vi "Curtin_SaveToExcel.vi"(8 "plots":refnum<vi>[](array[refnum])) -> ()   [LabVIEW 2022 SP3]
uses:
  <vilib>/express/express shared/NI_ExcelFile/Ctrls/FileOperation.ctl
  <vilib>/express/express shared/NI_ExcelFile/SubVIs/WriteData (Array of STR).vi
  <vilib>/express/express shared/NI_ExcelFile/NI_ExcelFile.lvlib
panel:
  in  "Average FRF 3":cluster{dbl, "df":dbl, dbl[]}[](graph)
  out "Average FRF 2":cluster{dbl, "df":dbl, dbl[]}[](graph)
  out "Average FRF":cluster{dbl, "df":dbl, dbl[]}[](graph)
  out "Breakdown":string[][](table)
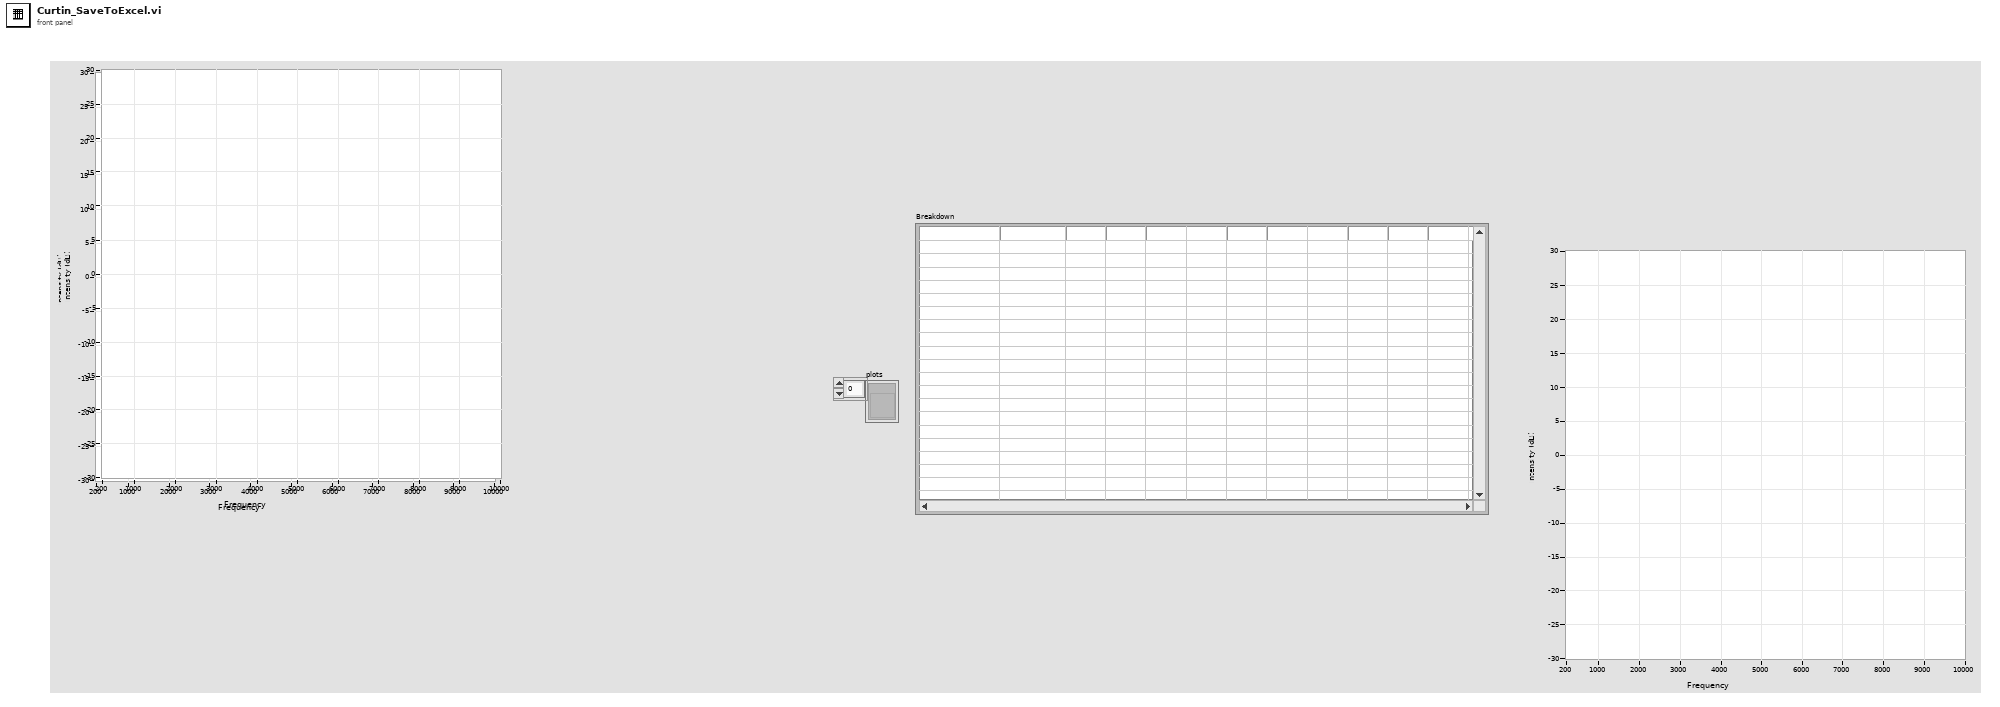
[diagram p1: front panel]
types:
  T1 = enum16{"Append values", "Create", "Replace values at index", "Replace all values"}
  T2 = typedef "NI_ExcelFile.lvlib/FileOperation.ctl" = enum16{"open or create", "open", "create or replace", "create"}
  T3 = typedef "NI_ExcelFile.lvlib/ExcelRefnum.ctl" = refnum<data-value>
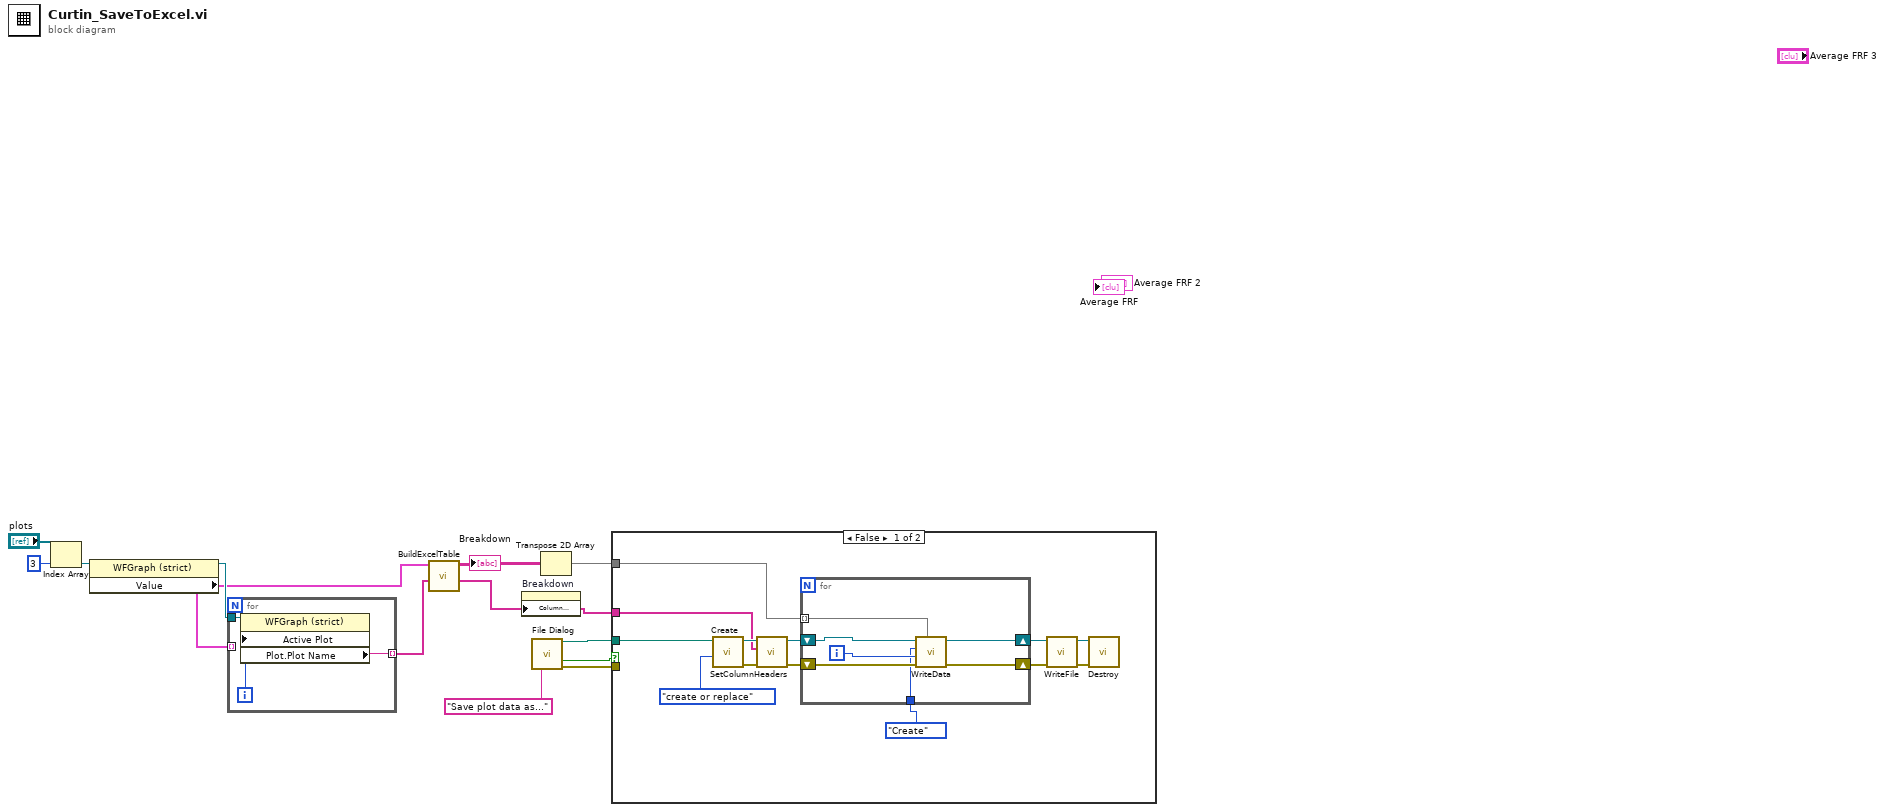
[diagram p0: block diagram]
diagram:
  n1 = Index Array(array="plots", index=3) -> (element=w7:refnum<vi>)
  n2 = property class="WFGraph (strict)"(reference=w7) -> (reference out=w6:refnum<vi>, "Value"=w5:cluster{dbl, "df":dbl, dbl[]}[])  [unwired: 1 in, 1 out]
  n3 = for {
    tunnel: w6 -> [w16]
    tunnel: w5 -> [_] mode=indexing
    tunnel: [w14] -> w4 mode=indexing
    i -> [w15]
    n4 = property class="WFGraph (strict)"(reference=w16, "Active Plot"=w15) -> ("Plot.Plot Name"=w14:string)  [unwired: 1 in, 2 out]
  }
  n5 = call "BuildExcelTable.vi"("Names"=w4, "Value"=w5) -> ("ColHeaders"=w10:string[], "Breakdown"=w9:string[][])  [unwired: 8 in]
  "Breakdown" <- w9
  n6 = property on="Breakdown" class="Tbl (strict)"("Column Headers[]"=w10) -> ()  [unwired: 2 in, 2 out]
  n7 = call "File Dialog"("prompt"="Save plot data as...") -> ("selected path"=w12:path, "cancelled"=w11:bool, "error out"=w2:errorcluster)  [unwired: 11 in, 1 out]
  n8 = Transpose 2D Array(2D array=w9) -> (transposed array=w13:string[][])
  n9 = case shown="False" w11 {
    tunnel: w13 -> [w21 _]
    tunnel: w10 -> [w20 _]
    tunnel: w12 -> [w19 _]
    tunnel: w2 -> [_ _]
    frame False {
      n10 = call <vilib>:"Create.vi"("operation (0: open or create)"=FileOperation."create or replace", "file"=w19) -> ("error out"=w24:errorcluster, "Excel refnum out"=w25:T3)  [unwired: 8 in]
      n11 = call <vilib>:"SetColumnHeaders.vi"("error in (no error)"=w24, "column headers"=w20, "Excel refnum"=w25) -> ("error out"=w28:errorcluster, "Excel refnum out"=w29:T3)  [unwired: 7 in]
      n12 = for {
        shift-right: [w36] -> w22
        shift-left: w28 -> [w34]
        shift-right: [w33] -> w23
        shift-left: w29 -> [w35]
        tunnel: w21 -> [w31] mode=indexing
        tunnel: T1."Create" ("operation (0: create)") -> [w30]
        i -> [w32]
        n13 = call-poly <vilib>:"WriteData.vi"("Array of STR"=w31, "error in (no error)"=w34, "channel index (0)"=w32, "operation (0: create)"=w30, "Excel refnum"=w35) -> ("error out"=w36:errorcluster, "Excel refnum out"=w33:T3)  [unwired: 5 in]
      }
      n14 = call <vilib>:"WriteFile.vi"("error in (no error)"=w22, "Excel refnum"=w23) -> ("error out"=w27:errorcluster, "Excel refnum out"=w26:T3)  [unwired: 8 in]
      n15 = call <vilib>:"Destroy.vi"("error in (no error)"=w27, "Excel refnum"=w26) -> ()  [unwired: 8 in, 2 out]
    }
    frame True {
    }
  }
